vi "Synchronize.vi"(7 "Retries":i32, 8 "Error In":errorcluster, 11 "LINX Device Config":T1) -> (0 "Error Out":errorcluster, 3 "LINX Device Config":T1)   [LabVIEW 2011, in "LVH-LINX.lvlib"]
doc: "Synchronize the LINX device with LabVIEW."
uses:
  LVH-LINX.lvlib
  Type Defs/LINX Device Config.ctl
  Type Defs/Interface.ctl
  Type Defs/TCP Config.ctl
  Error Type.ctl
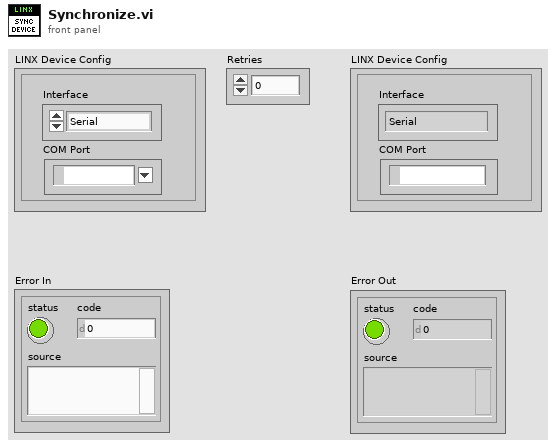
[diagram p1: front panel]
types:
  T1 = typedef "LVH-LINX.lvlib/LINX Device Config.ctl" = cluster{"Interface":T2, "COM Port":refnum<visa-resource-name>, "Packet Number":u16, "TCP Configuration":T3}
  T2 = typedef "LVH-LINX.lvlib/Interface.ctl" = enum16{"Serial", "TCP"}
  T3 = typedef "LVH-LINX.lvlib/TCP Config.ctl" = cluster{"IP Address":string, "Port":dbl}
  T4 = typedef "LVH-LINX.lvlib/Error Type.ctl" = enum16{"Unknown", "Timeout", "Corrupt Return Packet", "Unable To Connect"}
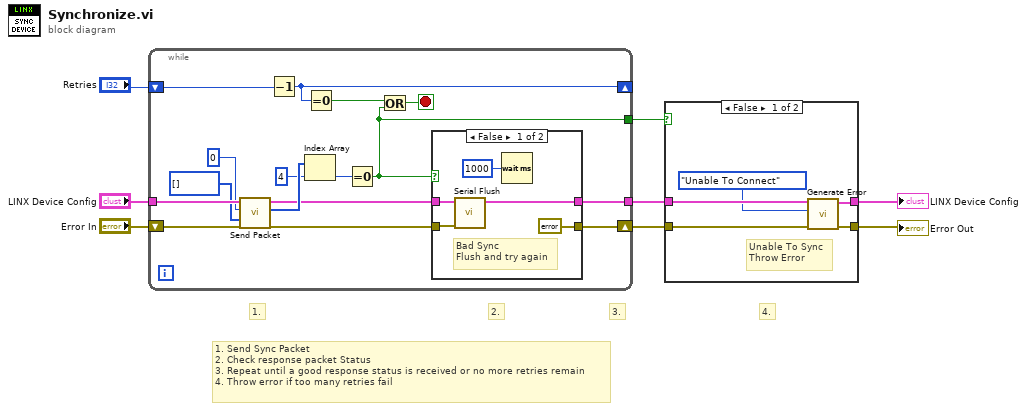
[diagram p0: block diagram]
diagram:
  # "4."
  # "3."
  # "2."
  # "1."
  # "1. Send Sync Packet\n2. Check response packet Status\n3. Repeat until a good response status is received or no more retries remain\n4. Throw error if too many retries fail"
  n1 = while {
    tunnel: "LINX Device Config" -> [w24]
    tunnel: [w14] -> w5
    shift-right: [w19] -> _
    shift-left: "Retries" -> [w20]
    shift-right: [w12] -> w4
    shift-left: "Error In" -> [w23]
    tunnel: [w9] -> w3
    stop <- w10 stop-if-true
    n2 = call "Send Packet.vi"("Error In"=w23, "ARGS"=u8[] [], "CMD"=u16 0, "LINX Device Config"=w24) -> ("Error Out"=w11:errorcluster, "Packet"=w18:u8[], "LINX Device Config"=w13:T1)  [unwired: 5 in]
    n3 = Decrement(x=w20) -> (x-1=w19:i32)
    n4 = Index Array(array=w18, index=4) -> (element=w16:u8)
    n5 = Equal To 0?(x=w19) -> (x = 0?=w15:bool)
    n6 = Equal To 0?(x=w16) -> (x = 0?=w9:bool)
    n7 = Or(x=w15, y=w9) -> (x .or. y?=w10:bool)
    n8 = case shown="False" w9 {
      tunnel: [w26 w31] -> w14
      tunnel: w13 -> [w29 w31]
      tunnel: [errorcluster {"status"=FALSE, "code"=0, "source"=""} ("Error Out") w30] -> w12
      tunnel: w11 -> [w28 w30]
      frame False {
        # "Bad Sync\nFlush and try again"
        n9 = call "Serial Flush.vi"("Error In"=w28, "LINX Device Config"=w29) -> ("LINX Device Config"=w26:T1)  [unwired: 8 in, 1 out]
        n10 = Wait (ms)(milliseconds to wait=u32 1000) -> ()  [unwired: 1 out]
      }
      frame True {
        # "Sync OK"
      }
    }
  }
  n11 = case shown="False" w3 {
    tunnel: [w36 w38] -> w2
    tunnel: w5 -> [w34 w38]
    tunnel: [w35 w37] -> w1
    tunnel: w4 -> [w32 w37]
    frame False {
      # "Unable To Sync\nThrow Error"
      n12 = call "Generate Error.vi"("Error In"=w32, "Error Type"=Error_Type."Unable To Connect", "LINX Device Config"=w34) -> ("Error Out"=w35:errorcluster, "LINX Device Config"=w36:T1)  [unwired: 7 in]
    }
    frame True {
      # "Sync OK"
    }
  }
  "Error Out" <- w1
  "LINX Device Config" <- w2
